vi "INCERTEZZA.vi"(4 "Cluster COLORS":cluster{"fore":u32, "back ER":u32, "back":u32}={"fore"=10197915, "back ER"=11796480, "back"=43}, 6 "NM?":bool, 7 "Array":T1(array[ring]), 8 "PDiff?":bool, 9 "Cluster INFO":T2={"Coefficenti P2"={"Af"=0.0, "Bf"=0.0, "Cf"=0.0, "Df"=0.0, "Ef"=0.0, "Ff"=0.0, "Gf"=0.0, "Hf"=0.0, "Jf"=0.0, "Kf"=0.0, "If"=0.0, "Ar"=0.0, "Br"=0.0, "Cr"=0.0, "Dr"=0.0, "Er"=0.0, "Fr"=0.0, "Gr"=0.0, "Hr"=0.0, "Jr"=0.0, "Kr"=0.0, "Ir"=0.0}, "Cluster settaggi wattmetro"={"Wattmetro"=enum."No Selection", "Alimentazione"=enum."Radio Selection 1"}, "SET RPM"=0.0, "SET TEMP"=0.0, "Costanti collaudo"={"P [bar]"=0.0, "T amb. [°C]"=0.0, "Umidità [%]"=0.0, "T acqua [°C] 2"=0.0}, "Condizione P2"=enum."Radio Selection 1", "Array linee"=[{"portata"=0, "Hasp"=0, "Hmand"=1, "Torsiometro"=0, "rpm"=0, "Hdiff?"=FALSE, "T amb"=0, "Indici valvole"=[0, 1], "Nome"="Elettropompa", "Sommersa?"=FALSE, "nomi valvole"=[]}, {"portata"=1, "Hasp"=0, "Hmand"=0, "Torsiometro"=0, "rpm"=0, "Hdiff?"=FALSE, "T amb"=0, "Indici valvole"=[0, 1], "Nome"="Sommersa", "Sommersa?"=TRUE, "nomi valvole"=[]}], "Array valvole linee avvio/fermata"=[], "Linea selezionata"=0.0, "Tolleranze croci"={"Q"=0.0, "Htot"=0.0, "Ptot"=0.0, "EtaP"=0.0}, "Sett T e R"={"Tamb[°C]"=0.0, "Ru-w"=0.0, "Rmarcia"=0.0, "Raux"=0.0, "Tamb Freddo[°C]"=0.0, "Ru-w freddo"=0.0, "Rmarcia freddo"=0.0, "Raux freddop"=0.0, "TC1"=0.0, "TC2"=0.0, "TC3"=0.0, "TC4"=0.0, "TC5"=0.0, "TC6"=0.0, "TC7"=0.0, "TC8"=0.0}, "Nomi valvole prop sistema"=[], "Calcolo P2"=enum."Torsiometro", "Rendimento motore"=0.0, "curva rendimento"=[], "Coeff motore"={"a6"=0.0, "a5"=0.0, "a4"=0.0, "a3"=0.0, "a2"=0.0, "a1"=0.0, "a0"=0.0, "P1max"=0.0, "P1min"=0.0}, "g[m/s2]"=0.0, "mandata"={"canale"="", "ai min"=0.0, "ai max"=0.0, "range"=0.0, "offset"=0.0, "UM"=enum."V"}, "aspirazione"={"canale"="", "ai min"=0.0, "ai max"=0.0, "range"=0.0, "offset"=0.0, "UM"=enum."V"}, "Array portate"=[], "canale-- sensore"=[], "SET Q A ZERO"={"Escludi lettura QDN25"=FALSE, "Escludi lettura QDN65"=FALSE}, "Premistoppa"={"canale"="", "ai min"=0.0, "ai max"=0.0, "range"=0.0, "offset"=0.0, "UM"=enum."V"}, "Prof.Vasca [m]"=0.0, "Offset sens liv[m]"=0.0, "Coppia"={"canale"="", "ai min"=0.0, "ai max"=0.0, "range"=0.0, "offset"=0.0, "UM"=enum."V"}, "Attriti B1"=[], "Attriti B2"=[]}, 10 "TABELLA risultati":refnum<vi>, 11 "TABELLA misure":refnum<vi>) -> (2 "ERROR":bool, 3 "riga aggiunta":string[](array[string]))   [LabVIEW 2016]
uses:
  TypeDef/Cluster INFO.ctl
  TypeDef/WT SELECTION.ctl
  TypeDef/ALIM SELECTION.ctl
  TypeDef/Definizione linea.ctl
  TypeDef/sett T e R.ctl
  formule.llb/Global.vi
panel:
  out "Array 2":T1(array[ring])
  # "Freddo"
  # "Regime"
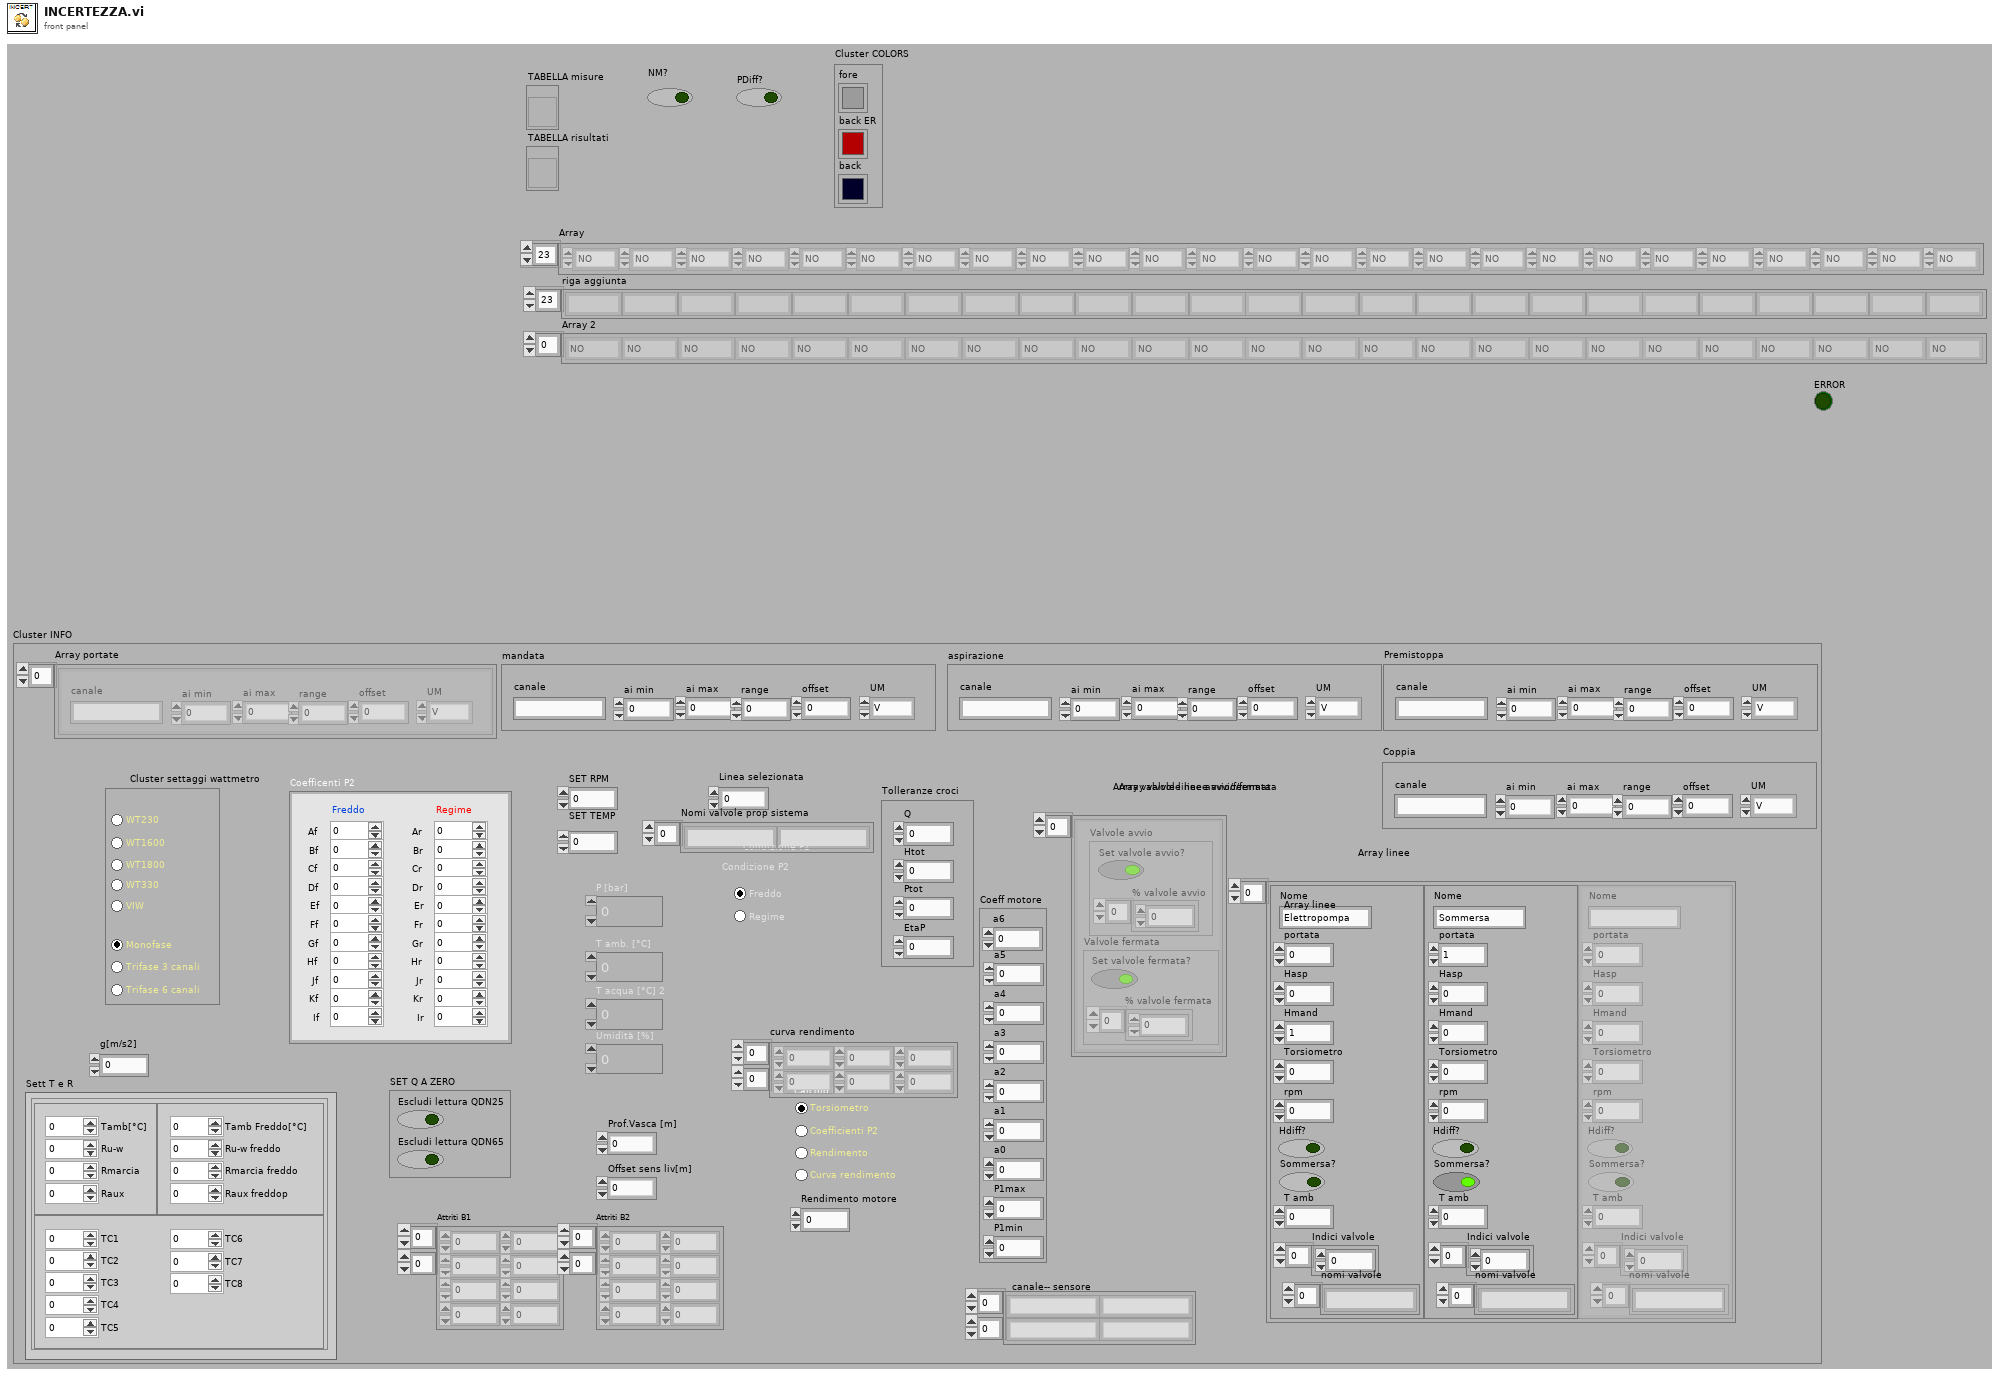
[diagram p1: front panel]
types:
  T1 = enum16{"NO", "Media", "Analisi", "Riporta primo"}[]
  T2 = typedef "Cluster INFO.ctl" = cluster{"Coefficenti P2":cluster{"Af":dbl, "Bf":dbl, "Cf":dbl, "Df":dbl, "Ef":dbl, "Ff":dbl, "Gf":dbl, "Hf":dbl, "Jf":dbl, "Kf":dbl, "If":dbl, "Ar":dbl, "Br":dbl, "Cr":dbl, "Dr":dbl, "Er":dbl, "Fr":dbl, "Gr":dbl, "Hr":dbl, "Jr":dbl, "Kr":dbl, "Ir":dbl}, "Cluster settaggi wattmetro":cluster{"Wattmetro":T3, "Alimentazione":T4}, "SET RPM":dbl, "SET TEMP":dbl, "Costanti collaudo":cluster{"P [bar]":dbl, "T amb. [°C]":dbl, "Umidità [%]":dbl, "T acqua [°C] 2":dbl}, "Condizione P2":enum32{"Radio Selection 1", "Radio Selection 2"}, "Array linee":T5[], "Array valvole linee avvio/fermata":cluster{"Valvole avvio":cluster{"Set valvole avvio?":bool, "% valvole avvio":dbl[]}, "Valvole fermata":cluster{"Set valvole fermata?":bool, "% valvole fermata":dbl[]}}[], "Linea selezionata":dbl, "Tolleranze croci":cluster{"Q":dbl, "Htot":dbl, "Ptot":dbl, "EtaP":dbl}, "Sett T e R":T6, "Nomi valvole prop sistema":string[], "Calcolo P2":enum32{"Torsiometro", "coeff p2", "Rendimento", "Curva rend"}, "Rendimento motore":dbl, "curva rendimento":dbl[][], "Coeff motore":cluster{"a6":dbl, "a5":dbl, "a4":dbl, "a3":dbl, "a2":dbl, "a1":dbl, "a0":dbl, "P1max":dbl, "P1min":dbl}, "g[m/s2]":dbl, "mandata":cluster{"canale":string, "ai min":dbl, "ai max":dbl, "range":dbl, "offset":dbl, "UM":T7}, "aspirazione":cluster{"canale":string, "ai min":dbl, "ai max":dbl, "range":dbl, "offset":dbl, "UM":T7}, "Array portate":cluster{"canale":string, "ai min":dbl, "ai max":dbl, "range":dbl, "offset":dbl, "UM":T7}[], "canale-- sensore":string[][], "SET Q A ZERO":cluster{"Escludi lettura QDN25":bool, "Escludi lettura QDN65":bool}, "Premistoppa":cluster{"canale":string, "ai min":dbl, "ai max":dbl, "range":dbl, "offset":dbl, "UM":T7}, "Prof.Vasca [m]":dbl, "Offset sens liv[m]":dbl, "Coppia":cluster{"canale":string, "ai min":dbl, "ai max":dbl, "range":dbl, "offset":dbl, "UM":T7}, "Attriti B1":dbl[][], "Attriti B2":dbl[][]}
  T3 = typedef "WT SELECTION.ctl" = enum32{"No Selection", "WT230", "WT1600", "WT1800", "WT330", "VIW"}
  T4 = typedef "ALIM SELECTION.ctl" = enum32{"Radio Selection 1", "Radio Selection 2", "Radio Selection 3"}
  T5 = typedef "Definizione linea.ctl" = cluster{"portata":i32, "Hasp":i32, "Hmand":i32, "Torsiometro":i32, "rpm":i32, "Hdiff?":bool, "T amb":i32, "Indici valvole":i16[], "Nome":string, "Sommersa?":bool, "nomi valvole":string[]}
  T6 = typedef "sett T e R.ctl" = cluster{"Tamb[°C]":dbl, "Ru-w":dbl, "Rmarcia":dbl, "Raux":dbl, "Tamb Freddo[°C]":dbl, "Ru-w freddo":dbl, "Rmarcia freddo":dbl, "Raux freddop":dbl, "TC1":dbl, "TC2":dbl, "TC3":dbl, "TC4":dbl, "TC5":dbl, "TC6":dbl, "TC7":dbl, "TC8":dbl}
  T7 = typedef "UnitàMisura.ctl" = enum16{"V", "mA", "Bar", "RPM", "m3/s", "m3/min", "m3/h", "l/s", "l/min", "in3/min", "ft3/min", "gpm", "igpm", "igph", "%", "°C", "m", "Nm"}
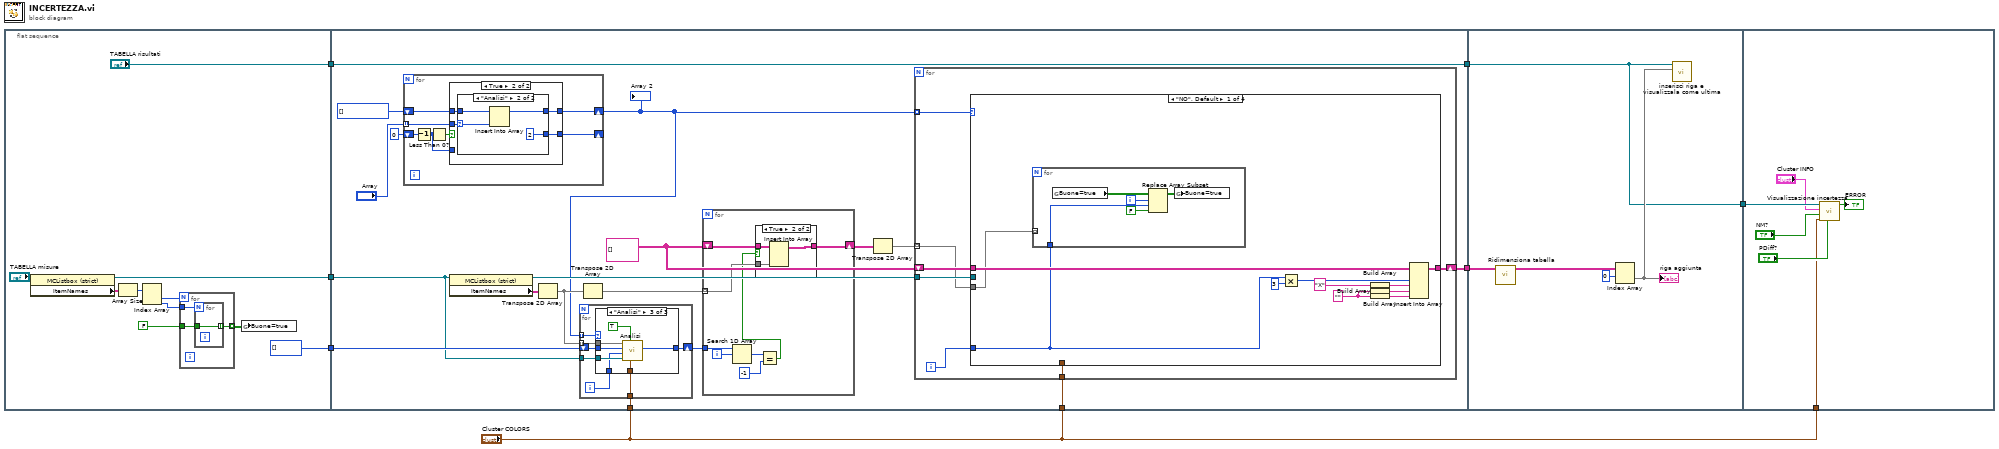
[diagram p0: block diagram]
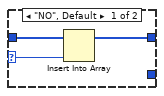
[diagram p3: hidden frame]
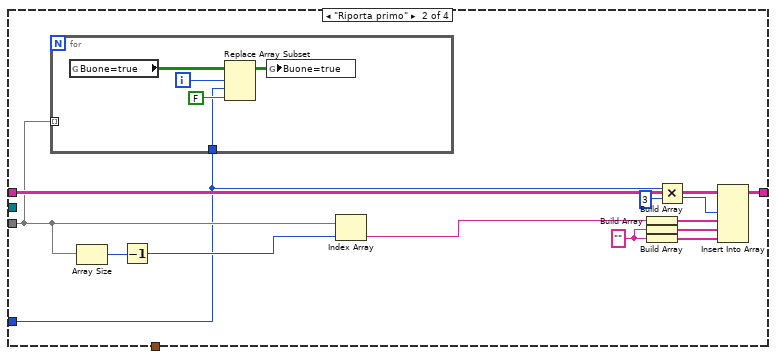
[diagram p7: hidden frame]
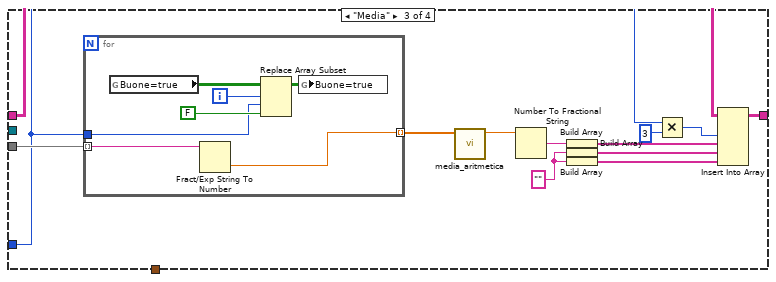
[diagram p8: hidden frame]
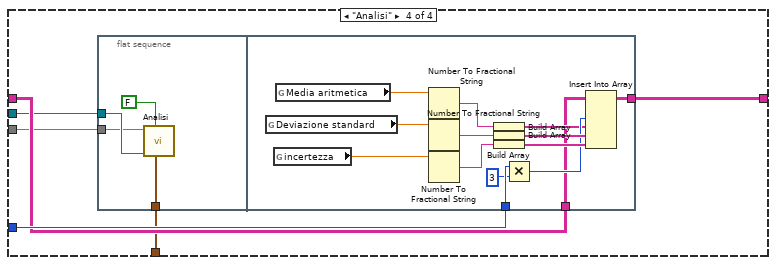
[diagram p9: hidden frame]
diagram:
  n1 = flat-sequence {
    tunnel: [w14] -> w6
    tunnel: ["TABELLA risultati"] -> w4
    tunnel: [i32[] [] ("Array index eliminati in")] -> w3
    tunnel: [w39] -> w7
    tunnel: w6 -> [w34]
    tunnel: [w37] -> w5
    tunnel: w4 -> [w37]
    tunnel: w3 -> [w35]
    tunnel: "Cluster COLORS" -> [w27]
    tunnel: "Cluster COLORS" -> [w26]
    tunnel: w7 -> [w177]
    tunnel: w5 -> [w173]
    tunnel: [w173] -> w2
    tunnel: w2 -> [w183]
    tunnel: "Cluster COLORS" -> [w179]
    frame #0 {
      n2 = property class="MCListbox (strict)"(reference="TABELLA misure") -> (reference out=w14:refnum<vi>, "ItemNames"=w15:string[][])  [unwired: 1 in, 1 out]
      n3 = Array Size(array=w15) -> (size(s)=w13:i32[])
      n4 = Index Array(array=w13) -> (element #1=w11:i32, element #2=w12:i32)  [unwired: 2 in]
      n5 = for {
        N: w11 -> [_]
        tunnel: [w20] -> w16 mode=indexing
        tunnel: FALSE -> [w19]
        tunnel: w12 -> [w18]
        n6 = for {
          N: w18 -> [_]
          tunnel: [w21] -> w20 mode=indexing
          tunnel: w19 -> [w21]
        }
      }
      n7 = global write "Global.vi" "Buone=true"(w16) -> ()
    }
    frame #1 {
      w24 = T1 [] items=["NO", "Media", "Analisi", "Riporta primo"] ("Array")
      w28 = string[][] []
      n8 = for {
        shift-right: [w44] -> w23
        shift-left: w24 -> [w46]
        tunnel: "Array" -> [w45] mode=indexing
        shift-right: [w43] -> _
        shift-left: 0 -> [w42]
        n9 = Decrement(x=w42) -> (x-1=w40:i32)
        n10 = Less Than 0?(x=w40) -> (x < 0?=w41:bool)
        n11 = case shown="True" w41 {
          tunnel: w46 -> [w47 w52]
          tunnel: w45 -> [_ w51]
          tunnel: [w47 w50] -> w44
          tunnel: [w48 w49] -> w43
          tunnel: w40 -> [w48 _]
          frame False {
          }
          frame True {
            n12 = case shown="\"Analisi\"" w51 {
              selector: w51 -> [w54 w58]
              tunnel: w52 -> [w55 w59]
              tunnel: [w53 w56] -> w50
              tunnel: [_ 2] -> w49
              frame "NO", Default {
                n13 = Insert Into Array(array=w55, new element=w54) -> (w53:T1)  [unwired: 1 in]
              }
              frame "Analisi" {
                n14 = Insert Into Array(array=w59, new element=w58) -> (w56:T1)  [unwired: 1 in]
              }
            }
          }
        }
      }
      "Array 2" <- w23
      n15 = property class="MCListbox (strict)"(reference=w34) -> (reference out=w36:refnum<vi>, "ItemNames"=w38:string[][])  [unwired: 1 in, 1 out]
      n16 = Transpose 2D Array(2D array=w38) -> (transposed array=w33:string[][])
      n17 = for {
        tunnel: w33 -> [w78] mode=indexing
        shift-right: [w77] -> w32
        shift-left: w35 -> [w76]
        tunnel: w23 -> [w75] mode=indexing
        tunnel: w34 -> [w74]
        tunnel: w27 -> [w72]
        i -> [w73]
        n18 = case shown="\"Analisi\"" w75 {
          tunnel: w78 -> [_ _ w87]
          tunnel: [w79 w80 w86] -> w77
          tunnel: w76 -> [w79 w80 w85]
          tunnel: w74 -> [_ _ w84]
          tunnel: w73 -> [_ _ w82]
          tunnel: w72 -> [_ _ w81]
          frame "NO", Default {
          }
          frame "Media" {
          }
          frame "Analisi" {
            n19 = call "Analisi.vi"("Cluster COLORS"=w81, "crea\ntabella scarti"=TRUE ("bypass\ntabella scarti"), "MCListbox tabella dati"=w84, "n colonna"=w82, "Array index eliminati in"=w85, "Array"=w87) -> ("Array index eliminati"=w86:i32[])  [unwired: 5 out]
          }
        }
      }
      n20 = Transpose 2D Array(2D array=w33) -> (transposed array=w31:string[][])
      n21 = for {
        tunnel: w32 -> [w66]
        tunnel: w31 -> [w64] mode=indexing
        shift-right: [w60] -> w30
        shift-left: w28 -> [w65]
        i -> [w67]
        n22 = Search 1D Array(1D array=w66, element=w67) -> (index of element=w63:i32)  [unwired: 1 in]
        n23 = Equal?(x=w63, y=-1) -> (x = y?=w61:bool)
        n24 = case shown="True" w61 {
          tunnel: w65 -> [w68 w71]
          tunnel: w64 -> [_ w70]
          tunnel: [w68 w69] -> w60
          frame False {
          }
          frame True {
            n25 = Insert Into Array(array=w71, new element=w70) -> (w69:string[][])  [unwired: 2 in]
          }
        }
      }
      n26 = Transpose 2D Array(2D array=w30) -> (transposed array=w29:string[][])
      n27 = for {
        tunnel: w23 -> [w94] mode=indexing
        shift-right: [w92] -> w39
        shift-left: w28 -> [w93]
        tunnel: w36 -> [w90]
        tunnel: w29 -> [w89] mode=indexing
        tunnel: w26 -> [w88]
        i -> [w91]
        n28 = case shown="\"NO\", Default" w94 {
          tunnel: w89 -> [w96 w114 w141 w150]
          tunnel: w91 -> [w95 w111 w129 w154]
          tunnel: w93 -> [w99 w117 w131 w153]
          tunnel: [w98 w116 w130 w152] -> w92
          tunnel: w90 -> [_ _ _ w151]
          tunnel: w88 -> [_ _ _ w149]
          frame "NO", Default {
            w102 = ""
            n29 = for {
              tunnel: w96 -> [_] mode=indexing
              tunnel: w95 -> [w106]
              i -> [w107]
              n30 = global read "Global.vi" "Buone=true"() -> (w110:bool[][])
              n31 = Replace Array Subset(array=w110, new element=FALSE ("Boolean"), index (row)=w107, index (col)=w106) -> (w109:bool[][])
              n32 = global write "Global.vi" "Buone=true"(w109) -> ()
            }
            n33 = Multiply(x=w95, y=3) -> (x*y=w104:i32)
            n34 = Build Array("X" ("element")) -> (w103:string[])
            n35 = Build Array(w102) -> (w101:string[])
            n36 = Build Array(w102) -> (w100:string[])
            n37 = Insert Into Array(array=w99, index (col)=w104, new element #1=w103, new element #2=w101, new element #3=w100) -> (w98:string[][])  [unwired: 1 in]
          }
          frame "Riporta primo" {
            w120 = ""
            n38 = for {
              tunnel: w114 -> [_] mode=indexing
              tunnel: w111 -> [w124]
              i -> [w125]
              n39 = global read "Global.vi" "Buone=true"() -> (w128:bool[][])
              n40 = Replace Array Subset(array=w128, new element=FALSE ("Boolean"), index (row)=w125, index (col)=w124) -> (w127:bool[][])
              n41 = global write "Global.vi" "Buone=true"(w127) -> ()
            }
            n42 = Array Size(array=w114) -> (size(s)=w113:i32)
            n43 = Decrement(x=w113) -> (x-1=w112:i32)
            n44 = Index Array(array=w114, index=w112) -> (element=w115:string)
            n45 = Build Array(w115) -> (w121:string[])
            n46 = Build Array(w120) -> (w119:string[])
            n47 = Build Array(w120) -> (w118:string[])
            n48 = Multiply(x=w111, y=3) -> (x*y=w122:i32)
            n49 = Insert Into Array(array=w117, index (col)=w122, new element #1=w121, new element #2=w119, new element #3=w118) -> (w116:string[][])  [unwired: 1 in]
          }
          frame "Media" {
            w134 = ""
            n50 = for {
              tunnel: w141 -> [w148] mode=indexing
              tunnel: [w147] -> w140 mode=indexing
              tunnel: w129 -> [w142]
              i -> [w143]
              n51 = global read "Global.vi" "Buone=true"() -> (w146:bool[][])
              n52 = Fract/Exp String To Number(string=w148) -> (number=w147:dbl)  [unwired: 4 out]
              n53 = Replace Array Subset(array=w146, new element=FALSE ("Boolean"), index (row)=w143, index (col)=w142) -> (w145:bool[][])
              n54 = global write "Global.vi" "Buone=true"(w145) -> ()
            }
            n55 = call "media_aritmetica.vi"("Array"=w140) -> ("Media aritmetica"=w136:dbl)  [unwired: 10 out]
            n56 = Number To Fractional String(number=w136) -> (F-format string=w137:string)  [unwired: 3 out]
            n57 = Build Array(w137) -> (w135:string[])
            n58 = Build Array(w134) -> (w133:string[])
            n59 = Build Array(w134) -> (w132:string[])
            n60 = Multiply(x=w129, y=3) -> (x*y=w138:i32)
            n61 = Insert Into Array(array=w131, index (col)=w138, new element #1=w135, new element #2=w133, new element #3=w132) -> (w130:string[][])  [unwired: 1 in]
          }
          frame "Analisi" {
            n62 = flat-sequence {
              tunnel: w151 -> [w158]
              tunnel: w150 -> [w157]
              tunnel: w149 -> [w155]
              tunnel: w154 -> [w170]
              tunnel: w153 -> [w161]
              tunnel: [w160] -> w152
              frame #0 {
                n63 = call "Analisi.vi"("Cluster COLORS"=w155, "crea\ntabella scarti"=FALSE ("bypass\ntabella scarti"), "MCListbox tabella dati"=w158, "Array"=w157) -> ()  [unwired: 2 in, 6 out]
              }
              frame #1 {
                n64 = global read "Global.vi" "Deviazione standard"() -> (w165:dbl)
                n65 = global read "Global.vi" "incertezza"() -> (w159:dbl)
                n66 = global read "Global.vi" "Media aritmetica"() -> (w166:dbl)
                n67 = Number To Fractional String(number=w166) -> (F-format string=w164:string)  [unwired: 3 out]
                n68 = Number To Fractional String(number=w165) -> (F-format string=w163:string)  [unwired: 3 out]
                n69 = Number To Fractional String(number=w159) -> (F-format string=w162:string)  [unwired: 3 out]
                n70 = Build Array(w164) -> (w167:string[])
                n71 = Build Array(w163) -> (w172:string[])
                n72 = Build Array(w162) -> (w171:string[])
                n73 = Multiply(x=w170, y=3) -> (x*y=w168:i32)
                n74 = Insert Into Array(array=w161, index (col)=w168, new element #1=w167, new element #2=w172, new element #3=w171) -> (w160:string[][])  [unwired: 1 in]
              }
            }
          }
        }
      }
    }
    frame #2 {
      n75 = call "Ridimensiona tabella.vi"("Array"=w177) -> ("Array 2"=w176:string[][])  [unwired: 10 out]
      n76 = Index Array(array=w176, index (row)=0) -> (element=w174:string[])  [unwired: 1 in]
      "riga aggiunta" <- w174
      n77 = call <userlib>:"inserisci riga e visualizzala come ultima.vi"("new element/subarray"=w174, "MulticolumnListbox in"=w173) -> ()  [unwired: 7 in, 3 out]
    }
    frame #3 {
      n78 = call "Visualizzazione incertezza.vi"("PDiff?"="PDiff?", "Cluster COLORS"=w179, "NM?"="NM?", "Cluster INFO"="Cluster INFO", "MCListbox Refnum"=w183) -> ("ERROR"=→"ERROR":bool)  [unwired: 6 in]
    }
  }
